vi "数字键盘.vi"(1 "显示样式":u32, 2 "OldNumber":dbl) -> (0 "NewNumber":dbl)   [LabVIEW 2016, in "斯坦道多参数.lvlib"]
panel:
  in  "数值":dbl
  in  "OK Button":bool
  in  "Cancel":bool
  in  "OK":bool
  in  "Clear":bool
  in  "BackSpace":bool
  in  "String":string
  in  "Point":bool
  in  "Zero":bool
  in  "Nine":bool
  in  "Eight":bool
  in  "Seven":bool
  in  "Six":bool
  in  "Five":bool
  in  "Four":bool
  in  "Three":bool
  in  "Two":bool
  in  "One":bool
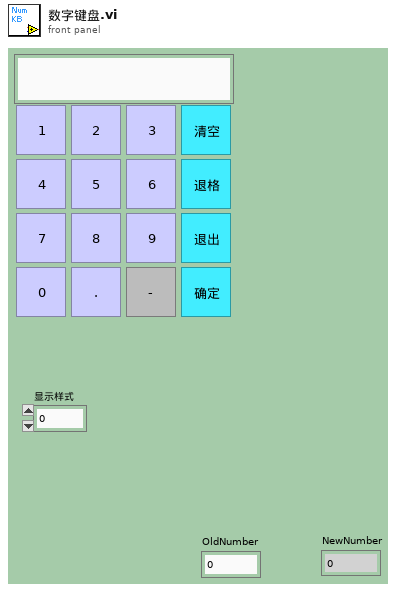
[diagram p1: front panel]
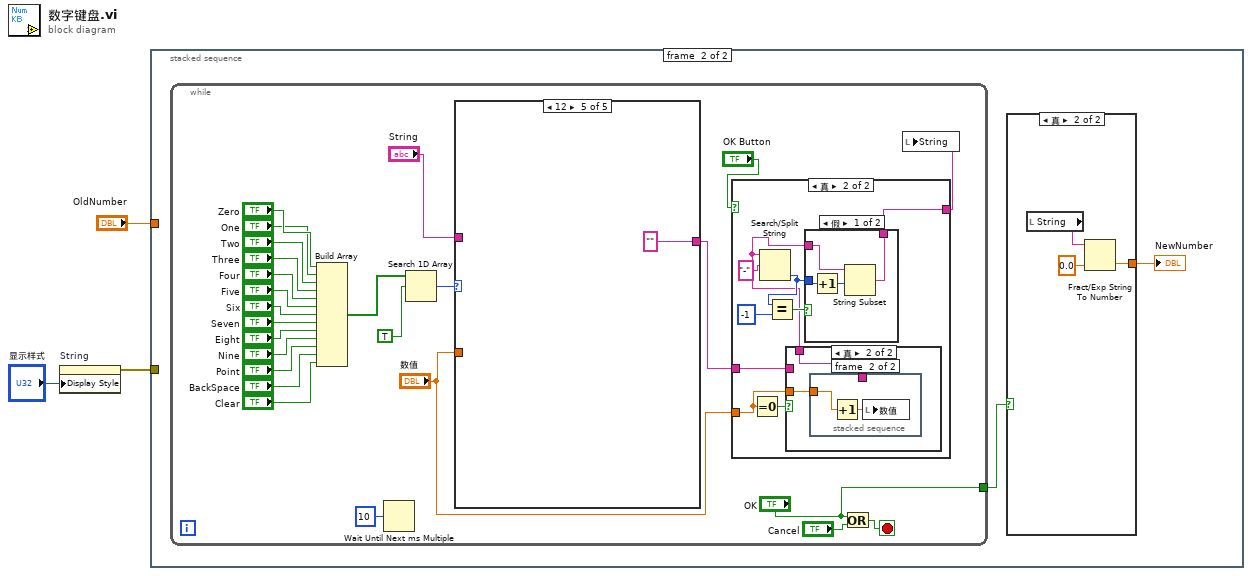
[diagram p0: block diagram]
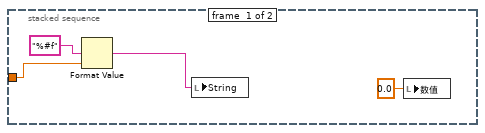
[diagram p2: hidden frame]
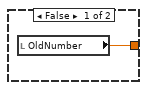
[diagram p3: hidden frame]
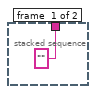
[diagram p6: hidden frame]
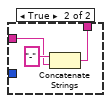
[diagram p7: hidden frame]
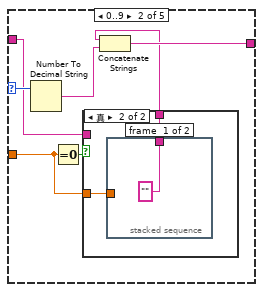
[diagram p9: hidden frame]
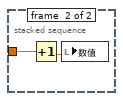
[diagram p11: hidden frame]
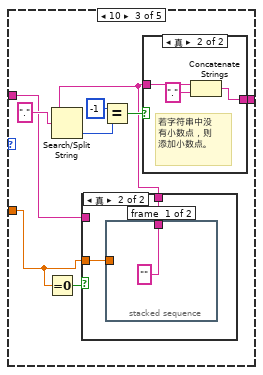
[diagram p12: hidden frame]
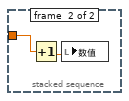
[diagram p14: hidden frame]
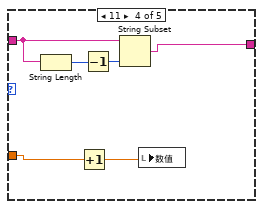
[diagram p16: hidden frame]
diagram:
  n1 = property on="String" class="Str"("Display Style"="显示样式") -> (error out=w2:errorcluster)  [unwired: 2 in, 1 out]
  n2 = stacked-sequence {
    tunnel: "OldNumber" -> [w4 _]
    tunnel: w2 -> [_ _]
    frame #0 {
      n3 = Format Value(format string="%#f" ("格式字符串"), value (0)=w4) -> (output string=w5:string)  [unwired: 1 in]
      n4 = local write "String"(w5) -> ()
      n5 = local write "数值"(0.0 ("数值")) -> ()
    }
    frame #1 {
      n6 = while {
        tunnel: ["OK"] -> w9
        stop <- w37 stop-if-true
        n7 = Build Array("Zero", "One", "Two", "Three", "Four", "Five", "Six", "Seven", "Eight", "Nine", "Point", "BackSpace", "Clear") -> (w22:bool[])
        n8 = Wait Until Next ms Multiple(millisecond multiple=u32 10) -> ()  [unwired: 1 out]
        n9 = Search 1D Array(1D array=w22, element=TRUE) -> (index of element=w20:i32)  [unwired: 1 in]
        n10 = case shown="12" w20 {
          selector: w20 -> [_ w69 _ _ _]
          tunnel: "String" -> [w62 w64 w79 w99 _]
          tunnel: [w62 w67 w80 w97 "" ("String")] -> w14
          tunnel: "数值" -> [_ w63 w76 w96 _]
          frame Default {
          }
          frame 0..9 {
            n11 = Number To Decimal String(number=w69) -> (decimal integer string=w68:string)  [unwired: 1 in]
            n12 = Equal To 0?(x=w63) -> (x = 0?=w66:bool)
            n13 = case shown="真" w66 {
              tunnel: [w70 w72] -> w65
              tunnel: w63 -> [_ w71]
              tunnel: w64 -> [w70 _]
              frame False {
              }
              frame True {
                n14 = stacked-sequence {
                  tunnel: ["" _] -> w72
                  tunnel: w71 -> [_ w75]
                  frame #0 {
                  }
                  frame #1 {
                    n15 = Increment(x=w75) -> (x+1=w74:dbl)
                    n16 = local write "数值"(w74) -> ()
                  }
                }
              }
            }
            n17 = Concatenate Strings(w65, w68) -> (w67:string)
          }
          frame 10 {
            n18 = Equal To 0?(x=w76) -> (x = 0?=w78:bool)
            n19 = case shown="真" w78 {
              tunnel: [w85 w87] -> w77
              tunnel: w79 -> [w85 _]
              tunnel: w76 -> [_ w86]
              frame False {
              }
              frame True {
                n20 = stacked-sequence {
                  tunnel: ["" _] -> w87
                  tunnel: w86 -> [_ w89]
                  frame #0 {
                  }
                  frame #1 {
                    n21 = Increment(x=w89) -> (x+1=w90:dbl)
                    n22 = local write "数值"(w90) -> ()
                  }
                }
              }
            }
            n23 = Search/Split String(string=w77, search string/char (-)=".") -> (offset of match=w83:i32)  [unwired: 1 in, 2 out]
            n24 = Equal?(x=-1, y=w83) -> (x = y?=w81:bool)
            n25 = case shown="真" w81 {
              tunnel: w77 -> [w91 w94]
              tunnel: [w91 w92] -> w80
              frame False {
              }
              frame True {
                # "若字符串中没\n有小数点，则\n添加小数点。"
                n26 = Concatenate Strings(w94, "." ("string")) -> (w92:string)
              }
            }
          }
          frame 11 {
            n27 = String Length(string=w99) -> (length=w98:i32)
            n28 = Increment(x=w96) -> (x+1=w95:dbl)
            n29 = Decrement(x=w98) -> (x-1=w100:i32)
            n30 = String Subset(string=w99, length (rest)=w100) -> (substring=w97:string)  [unwired: 1 in]
            n31 = local write "数值"(w95) -> ()
          }
          frame 12 {
          }
        }
        n32 = case shown="真" "OK Button" {
          tunnel: [w39 w45] -> w17
          tunnel: "数值" -> [_ w42]
          tunnel: w14 -> [w39 w41]
          frame False {
          }
          frame True {
            n33 = Equal To 0?(x=w42) -> (x = 0?=w43:bool)
            n34 = case shown="真" w43 {
              tunnel: [w49 w51] -> w40
              tunnel: w42 -> [_ w50]
              tunnel: w41 -> [w49 _]
              frame False {
              }
              frame True {
                n35 = stacked-sequence {
                  tunnel: ["" _] -> w51
                  tunnel: w50 -> [_ w53]
                  frame #0 {
                  }
                  frame #1 {
                    n36 = Increment(x=w53) -> (x+1=w54:dbl)
                    n37 = local write "数值"(w54) -> ()
                  }
                }
              }
            }
            n38 = Search/Split String(string=w40, search string/char (-)="-" ("搜索字符串/字符(-)")) -> (offset of match=w44:i32)  [unwired: 1 in, 2 out]
            n39 = Equal?(x=w44, y=-1) -> (x = y?=w46:bool)
            n40 = case shown="假" w46 {
              tunnel: w40 -> [w58 w60]
              tunnel: [w57 w59] -> w45
              tunnel: w44 -> [w56 _]
              frame False {
                n41 = Increment(x=w56) -> (x+1=w55:i32)
                n42 = String Subset(string=w58, offset (0)=w55) -> (substring=w57:string)  [unwired: 1 in]
              }
              frame True {
                n43 = Concatenate Strings("-" ("string"), w60) -> (w59:string)
              }
            }
          }
        }
        n44 = Or(x="OK", y="Cancel") -> (x .or. y?=w37:bool)
        n45 = local write "String"(w17) -> ()
      }
      n46 = case shown="真" w9 {
        tunnel: [w10 w11] -> w8
        frame False {
          n47 = local read "OldNumber"() -> (w10:dbl)
        }
        frame True {
          n48 = local read "String"() -> (w13:string)
          n49 = Fract/Exp String To Number(string=w13, default (0 dbl)=0.0 ("default (0 DBL)")) -> (number=w11:dbl)  [unwired: 2 in, 1 out]
        }
      }
      "NewNumber" <- w8
    }
  }
